vi "Check Parameter Dimensions.vi"(3 "Data Cluster":T2) -> (0 "Size of Parameter arrays":T1, 1 "Correct Dimension?":bool)   [LabVIEW 2019]
uses:
  controls/UI Data.ctl
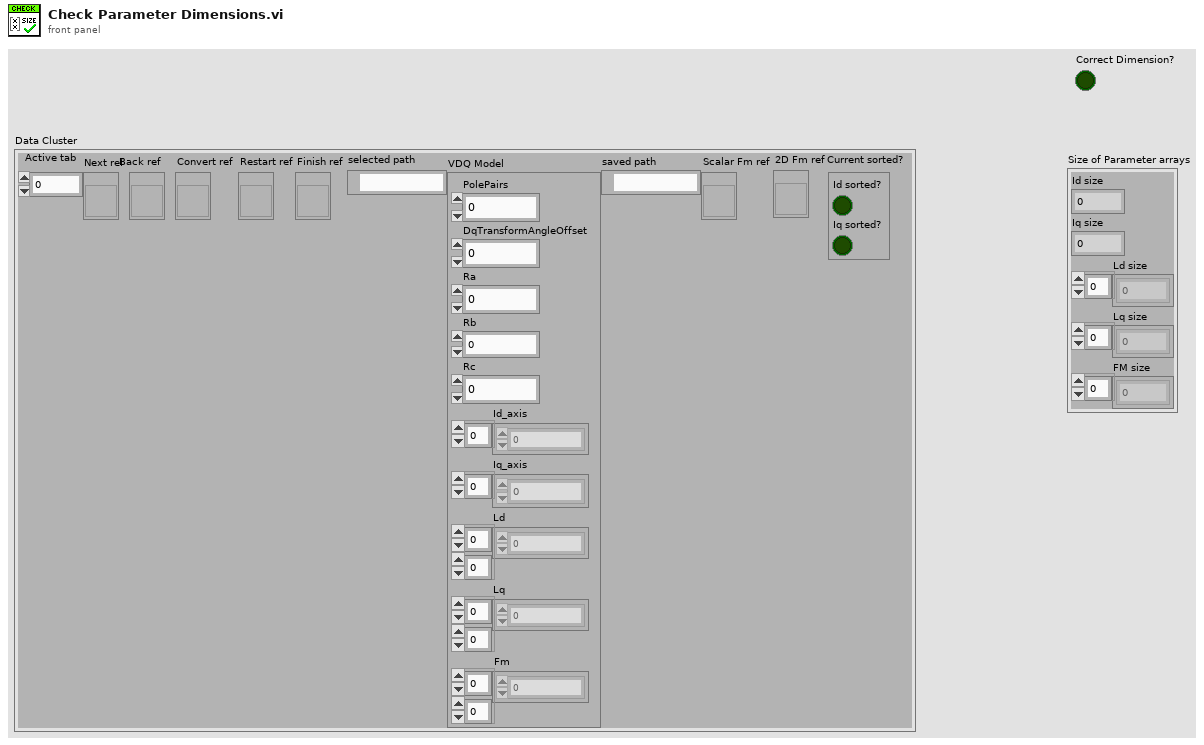
[diagram p1: front panel]
types:
  T1 = cluster{"Id size":i32, "Iq size":i32, "Ld size":i32[], "Lq size":i32[], "FM size":i32[]}
  T2 = typedef "UI Data.ctl" = cluster{"Active tab":u32, "Next ref":refnum<vi>, "Back ref":refnum<vi>, "Convert ref":refnum<vi>, "Restart ref":refnum<vi>, "Finish ref":refnum<vi>, "selected path":path, "VDQ Model":cluster{"PolePairs":dbl, "DqTransformAngleOffset":dbl, "Ra":dbl, "Rb":dbl, "Rc":dbl, "Id_axis":dbl[], "Iq_axis":dbl[], "Ld":dbl[][], "Lq":dbl[][], "Fm":dbl[][]}, "saved path":path, "Scalar Fm ref":refnum<vi>, "2D Fm ref":refnum<vi>, "Current sorted?":cluster{"Id sorted?":bool, "Iq sorted?":bool}}
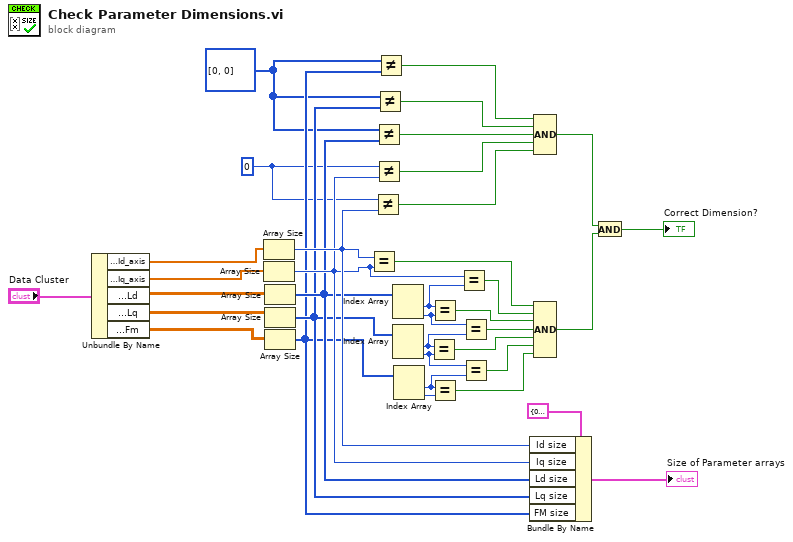
[diagram p0: block diagram]
diagram:
  w9 = 0 ("x")
  w10 = i32[] [0, 0] ("x")
  n1 = Unbundle By Name("Data Cluster") -> ("VDQ Model.Id_axis"=w20:dbl[], "VDQ Model.Iq_axis"=w19:dbl[], "VDQ Model.Ld"=w18:dbl[][], "VDQ Model.Lq"=w17:dbl[][], "VDQ Model.Fm"=w16:dbl[][])
  n2 = Array Size(array=w20) -> (size(s)=w15:i32)
  n3 = Array Size(array=w19) -> (size(s)=w14:i32)
  n4 = Array Size(array=w18) -> (size(s)=w13:i32[])
  n5 = Array Size(array=w17) -> (size(s)=w12:i32[])
  n6 = Array Size(array=w16) -> (size(s)=w11:i32[])
  n7 = Equal?(x=w15, y=w14) -> (x = y?=w36:bool)
  n8 = Not Equal?(x=w9, y=w15) -> (x != y?=w4:bool)
  n9 = Not Equal?(x=w10, y=w13) -> (x != y?=w6:bool)
  n10 = Not Equal?(x=w9, y=w14) -> (x != y?=w5:bool)
  n11 = Not Equal?(x=w10, y=w12) -> (x != y?=w7:bool)
  n12 = Not Equal?(x=w10, y=w11) -> (x != y?=w8:bool)
  n13 = Index Array(array=w13) -> (element #1=w29:i32, element #2=w25:i32)  [unwired: 2 in]
  n14 = Index Array(array=w12) -> (element #1=w26:i32, element #2=w27:i32)  [unwired: 2 in]
  n15 = Index Array(array=w11) -> (element #1=w28:i32, element #2=w24:i32)  [unwired: 2 in]
  n16 = Equal?(x=w26, y=w27) -> (x = y?=w31:bool)
  n17 = Equal?(x=w29, y=w25) -> (x = y?=w34:bool)
  n18 = Equal?(x=w28, y=w24) -> (x = y?=w33:bool)
  n19 = Equal?(x=w14, y=w29) -> (x = y?=w35:bool)
  n20 = Equal?(x=w25, y=w26) -> (x = y?=w30:bool)
  n21 = Equal?(x=w27, y=w28) -> (x = y?=w32:bool)
  n22 = Bundle By Name(cluster=T1 {"Id size"=0, "Iq size"=0, "Ld size"=[], "Lq size"=[], "FM size"=[]}, "Id size"=w15, "Iq size"=w14, "Ld size"=w13, "Lq size"=w12, "FM size"=w11) -> (→"Size of Parameter arrays":T1)
  n23 = Compound Arithmetic op=AND(w8, w7, w6, w5, w4) -> (w2:bool)
  n24 = Compound Arithmetic op=AND(w36, w35, w34, w30, w31, w32, w33) -> (w3:bool)
  n25 = And(x=w2, y=w3) -> (x .and. y?=→"Correct Dimension?":bool)
